vi "joinReadmodeNumber.vi"(2 "data in (U8) [0]":u8, 3 "read mode prefix [0:normal]":T1(ring)) -> (0 "data out (U32)":u32)   [LabVIEW 2015, in "Tausand AB1000.lvlib"]
doc: "Creates a number from the component bytes. \nMost significant byte: read mode.\n x0: normal read mode\n x1: crossed read, returns counters of a single channel \n (eg: A returns A, AB, AC, AD)\n x2: counters read (valid since AB2000 devices)\n x3: settings read (valid since AB2000 devices)\nLeast significant byte: data in (U8)."
uses:
  <instrlib>/Tausand AB1000/Tausand AB1000.lvlib
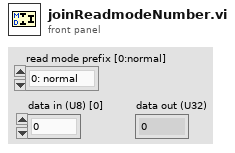
[diagram p1: front panel]
types:
  T1 = enum8{"0: normal", "1: channel", "2: all counters", "3: all settings"}
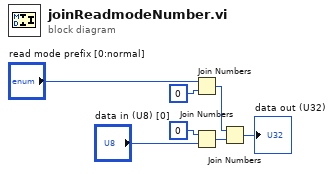
[diagram p0: block diagram]
diagram:
  n1 = Join Numbers(hi="read mode prefix [0:normal]", lo=u8 0 ("hi")) -> ((hi.lo)=w5:u16)
  n2 = Join Numbers(hi=u8 0, lo="data in (U8) [0]") -> ((hi.lo)=w4:u16)
  n3 = Join Numbers(hi=w5, lo=w4) -> ((hi.lo)=→"data out (U32)":u32)
